vi "TestJoystick.vi"() -> ()   [LabVIEW 2018]
uses:
  <vilib>/Rock Robotics/WPI/Joystick/WPI_JoystickDeviceEnum.ctl
  <vilib>/Rock Robotics/WPI/Utilities/WPI_GetSetVariantRefNum.vi
  <vilib>/Rock Robotics/WPI/Joystick/WPI_JoystickArcadeMapping.vi
panel:
  out "Right Motor Value":dbl
  out "Left Motor Value":dbl
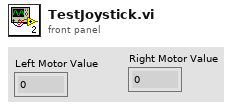
[diagram p1: front panel]
types:
  T1 = typedef "WPI_JoystickDeviceEnum.ctl" = enum16{"USB 0", "USB 1", "USB 2", "USB 3", "USB 4", "USB 5"}
  T2 = typedef "WPI_JoystickDevRef.ctl" = cluster{"Device":T1}
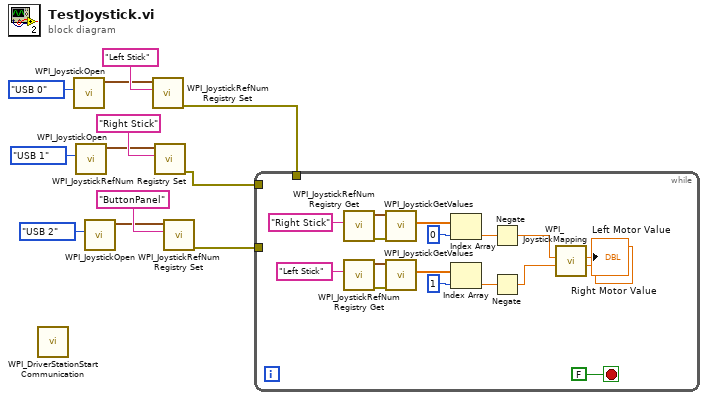
[diagram p0: block diagram]
diagram:
  n1 = call <vilib>:"WPI_DriverStationStart Communication.vi"() -> ()  [unwired: 12 in]
  n2 = call <vilib>:"WPI_JoystickOpen.vi"("JoystickDevice"=WPI_JoystickDeviceEnum."USB 0") -> ("JoystickDevRef"=w11:T2)  [unwired: 10 in]
  n3 = call <vilib>:"WPI_JoystickOpen.vi"("JoystickDevice"=WPI_JoystickDeviceEnum."USB 1") -> ("JoystickDevRef"=w8:T2)  [unwired: 10 in]
  n4 = call <vilib>:"WPI_JoystickOpen.vi"("JoystickDevice"=WPI_JoystickDeviceEnum."USB 2") -> ("JoystickDevRef"=w5:T2)  [unwired: 10 in]
  n5 = call <vilib>:"WPI_JoystickRefNum Registry Set.vi"("refnum name"="Left Stick", "JoystickDevRef"=w11) -> ("error out"=w3:errorcluster)  [unwired: 8 in, 1 out]
  n6 = call <vilib>:"WPI_JoystickRefNum Registry Set.vi"("refnum name"="Right Stick", "JoystickDevRef"=w8) -> ("error out"=w2:errorcluster)  [unwired: 8 in, 1 out]
  n7 = call <vilib>:"WPI_JoystickRefNum Registry Set.vi"("refnum name"="ButtonPanel", "JoystickDevRef"=w5) -> ("error out"=w1:errorcluster)  [unwired: 8 in, 1 out]
  n8 = while {
    tunnel: w3 -> [_]
    tunnel: w2 -> [_]
    tunnel: w1 -> [_]
    stop <- FALSE stop-if-true
    n9 = call <vilib>:"WPI_JoystickRefNum Registry Get.vi"("refnum name"="Right Stick") -> ("error out"=w24:errorcluster, "JoystickDevRef"=w25:T2)  [unwired: 9 in]
    n10 = call <vilib>:"WPI_JoystickRefNum Registry Get.vi"("refnum name"="Left Stick") -> ("error out"=w18:errorcluster, "JoystickDevRef"=w19:T2)  [unwired: 9 in]
    n11 = call <vilib>:"WPI_JoystickGetValues.vi"("error in (no error)"=w24, "JoystickDevRef"=w25) -> ("Axes"=w27:dbl[])  [unwired: 5 in, 4 out]
    n12 = call <vilib>:"WPI_JoystickGetValues.vi"("error in (no error)"=w18, "JoystickDevRef"=w19) -> ("Axes"=w22:dbl[])  [unwired: 5 in, 4 out]
    n13 = Index Array(array=w27, index=0) -> (element=w23:dbl)
    n14 = Index Array(array=w22, index=1) -> (element=w20:dbl)
    n15 = Negate(x=w23) -> (-x=w16:dbl)
    n16 = Negate(x=w20) -> (-x=w15:dbl)
    n17 = call-poly <vilib>:"WPI_JoystickMapping.vi"("Y axis value"=w15, "X axis value"=w16) -> ("Right Motor Value"=→"Right Motor Value":dbl, "Left Motor Value"=→"Left Motor Value":dbl)  [unwired: 8 in]
  }
